vi "Setting Keys.vi"() -> ()   [LabVIEW 2023, in "RFCalAndFixtureCharact.Common.lvlib"]
uses:
  RFCalAndFixtureCharact.Common.lvlib
panel:
  in  "CHARACTERIZE_BY_STANDARD":string="CharacterizeByStandard"
  in  "SIMULATED_POWER_METER_NAME":string="SimulatedPowerMeter"
  in  "POWER_METER_NAME":string="PowerMeterName"
  in  "OUTPUT_FOLDER_ABSOLUTE_PATH":string="OutputFolderAbsolutePath"
  in  "SIMULATION_ENABLED_FOR_OPERATOR_MODE":string="SimulationEnabledForOperatorMode"
  in  "CHARACT_TYPE":string="CharactType"
  in  "CHECK_PATH_EXPIRATION":string="CheckPathExpiration"
  in  "SILENT_OPTION_ENABLED":string="SilentOptionEnabled"
  in  "USE_OPERATOR_MODE":string="UseOperatorMode"
  in  "USE_COMMAND_LINE":string="UseCommandLine"
  in  "SEQUENCE_FILE_PATH":string="SequenceFilePath"
  in  "OUTPUT_FOLDER_RELATIVE_PATH":string="OutputFolderRelativePath"
  in  "CONFIG_FILE_RELATIVE_PATH":string="ConfigFileRelativePath"
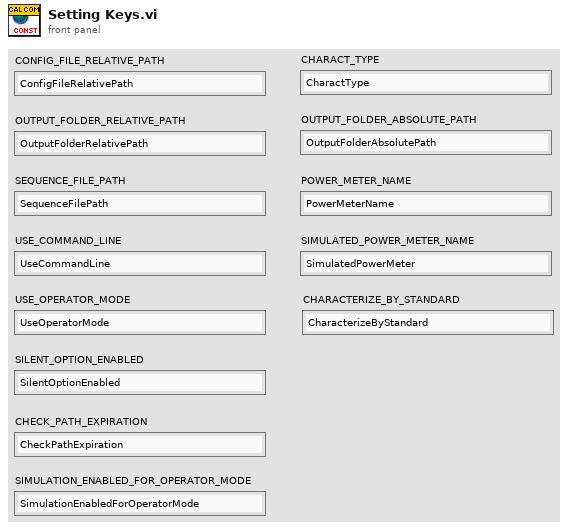
[diagram p1: front panel]
diagram:
